vi "Recieve server commands.vi"(8 "error in (no error)":errorcluster, 10 "bytes in":i64, 11 "Control-Client in":refnum<class "Control-Client.lvclass">) -> (0 "error out":errorcluster, 2 "bytes out":i64, 3 "Control-Client out":refnum<class "Control-Client.lvclass">)   [LabVIEW 2019, in "Control-Client.lvclass"]
uses:
  Control-Client.lvclass
  C:/Dev/TRANCON/Classes/GeneralFunctionality/GeneralFunctionality.lvclass
  dependecies/ControlsVIs/Clusters-def/Det-Reply-to-Read.ctl
  dependecies/ControlsVIs/Clusters-def/Def_signals_from_DET.ctl
  Control-Client.lvclass/Control-Client.ctl
  dependecies/ControlsVIs/Clusters-def/ProtypeCommand-CommandUnknown.ctl
  dependecies/ControlsVIs/Clusters-def/DL-Reply-to-Connect-to-Client.ctl
  dependecies/ControlsVIs/Clusters-def/Det-Reply-to-Connect-client.ctl
  dependecies/ControlsVIs/Clusters-def/DAQmx-Reply-Connect-client.ctl
  dependecies/ControlsVIs/Clusters-def/OSc-Reply-Connect-client.ctl
  dependecies/ControlsVIs/Clusters-def/CONTROL-Reply-Allconnect.ctl
  dependecies/ControlsVIs/Clusters-def/CONTROL-Reply-Status-client.ctl
  dependecies/ControlsVIs/Clusters-def/TEST-def.ctl
  dependecies/ControlsVIs/Clusters-def/DLMovedAxis-Com.ctl
  dependecies/ControlsVIs/Clusters-def/ProtypeCommand-DAQmxReply.ctl
  dependecies/ControlsVIs/Clusters-def/DAQmx-ELYSE_pulse_counter.ctl
  dependecies/ControlsVIs/Clusters-def/DAQmx-ELYSE_PumpSpeed.ctl
  dependecies/ControlsVIs/Clusters-def/OSc-Reply-Read.ctl
  dependecies/ControlsVIs/Clusters-def/Message types.ctl
  <vilib>/NI/STM/TCP/Read Message (TCP).vi
  <vilib>/NI/STM/NI STM.lvlib
  Message/Message.lvclass
  Delay Line/DelayLine.lvclass
  Detector/Detector.lvclass
  Control-Server/Control-Server.lvclass
  DAQmxTasks/DAQmxTaskContainer_General/DAQmxTaksContainer_General.lvclass
  Oscilloscope/Oscilloscope.lvclass
  GeneralFunctionality/GeneralFunctionality.lvclass
panel:
  in  "?":T1
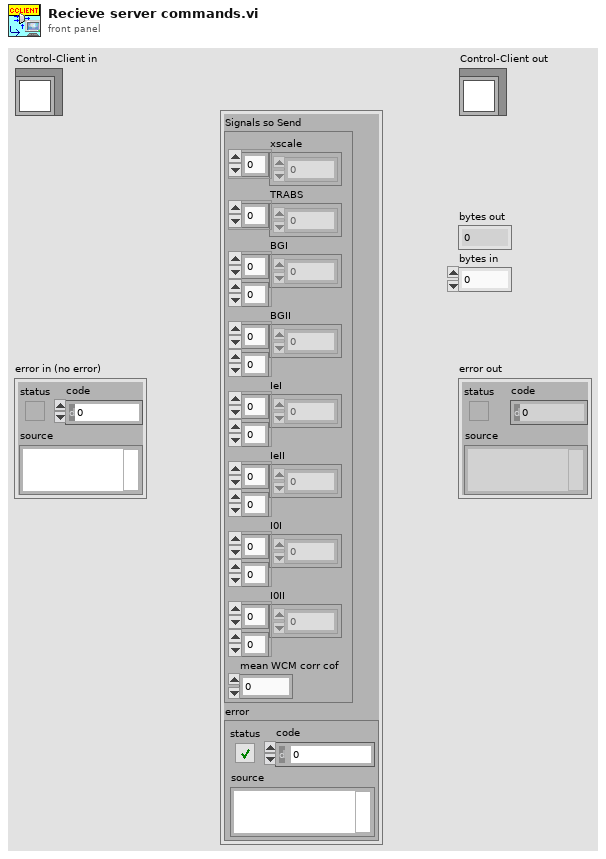
[diagram p1: front panel]
types:
  T1 = typedef "Detector.lvclass/Det-Reply-to-Read.ctl" = cluster{"Signals so Send":T2, "error":errorcluster}
  T2 = typedef "Detector.lvclass/Def_signals_from_DET.ctl" = cluster{"xscale":sgl[], "TRABS":sgl[], "BGI":sgl[][], "BGII":sgl[][], "IeI":sgl[][], "IeII":sgl[][], "I0I":sgl[][], "I0II":sgl[][], "mean WCM corr cof":dbl}
  T3 = typedef "ProtypeCommand-CommandUnknown.ctl" = cluster{"error in (no error)":errorcluster}
  T4 = typedef "DelayLine.lvclass/DL-Reply-to-Connect-to-Client.ctl" = cluster{"on/off":bool, "pos":dbl[], "param":cluster{"min":dbl, "max":dbl, "real pos":dbl}[], "predefine_pos":dbl[][], "error":errorcluster}
  T5 = typedef "Detector.lvclass/Det-Reply-to-Connect-client.ctl" = cluster{"on/off":bool, "calibration":dbl[], "error":errorcluster}
  T6 = typedef "DAQmxTaksContainer_General.lvclass/DAQmx-Reply-Connect-client.ctl" = cluster{"on/off":bool, "RelayKeyHeater/off":bool, "LaserShutter":bool, "AcceleratorShutter":bool, "Power":bool, "Faraday Cup Status":bool, "Pump Start_Stop":bool, "error":errorcluster}
  T7 = typedef "Oscilloscope.lvclass/OSc-Reply-Connect-client.ctl" = cluster{"on/off":bool, "WCM_state":bool, "error":errorcluster}
  T8 = typedef "Control-Server.lvclass/CONTROL-Reply-Allconnect.ctl" = cluster{"On/Off":bool, "error":errorcluster}
  T9 = typedef "Control-Client.lvclass/CONTROL-Reply-Status-client.ctl" = cluster{"DL reply to client":T4, "Det reply to client":cluster{"on/off":bool, "calibration":dbl[], "error out":errorcluster}, "DAQmx reply to client":T6, "OSc reply to CLIENT":T7}
  T10 = typedef "TEST-def.ctl" = cluster{"data":cluster{i32[], dbl[]}[]}
  T11 = typedef "DelayLine.lvclass/DLMovedAxis-Com.ctl" = cluster{"axis":i32, "what was asked":dbl, "where is is now":dbl, "Moved":bool, "error in (no error)":errorcluster}
  T12 = typedef "ProtypeCommand-DAQmxReply.ctl" = cluster{"On/Off":bool, "error out":errorcluster}
  T13 = typedef "DAQmxTaksContainer_General.lvclass/DAQmx-ELYSE_pulse_counter.ctl" = cluster{"# counts":dbl}
  T14 = typedef "DAQmxTaksContainer_General.lvclass/DAQmx-ELYSE_PumpSpeed.ctl" = cluster{"speed, rpm":dbl}
  T15 = typedef "Oscilloscope.lvclass/OSc-Reply-Read.ctl" = cluster{"Data":waveform(dbl)[], "Channels":u16[], "error":errorcluster}
  T16 = typedef "Message types.ctl" = string
  T17 = typedef "NI STM.lvlib/TCP Connection Info.ctl" = cluster{"connection ID":refnum<k5>, "meta data":T18[]}
  T18 = typedef "NI STM.lvlib/MetaDataElement.ctl" = string
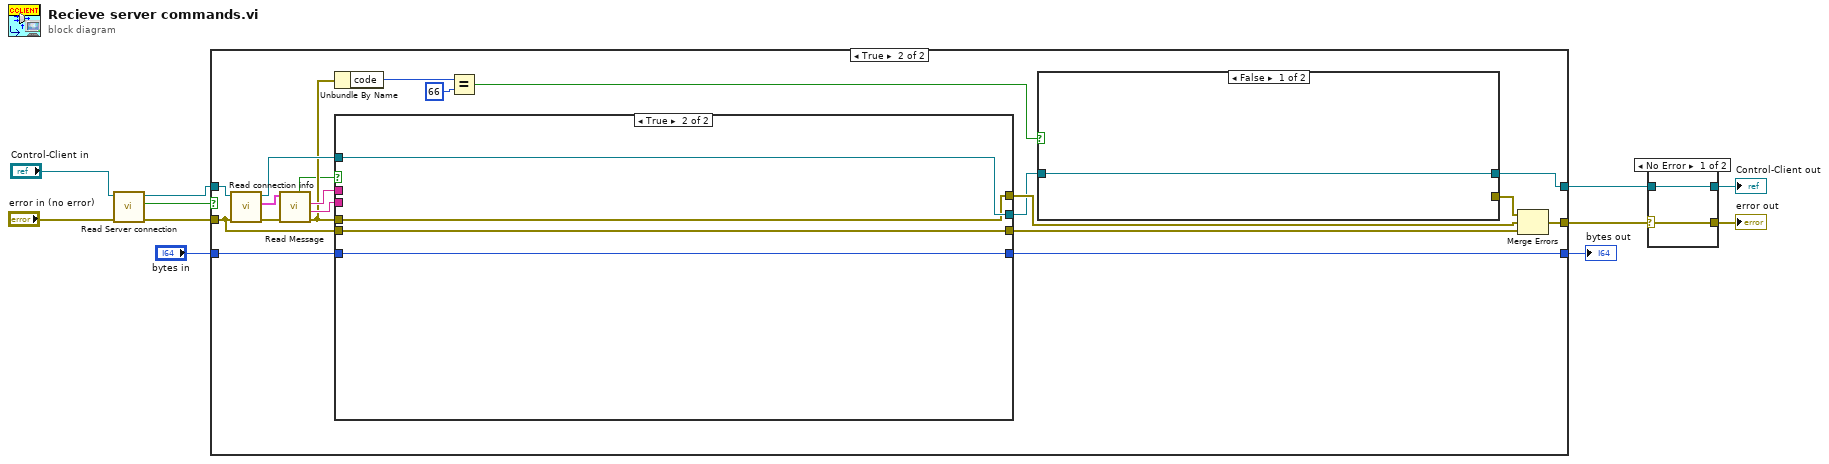
[diagram p0: block diagram]
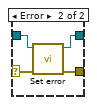
[diagram p2: hidden frame]
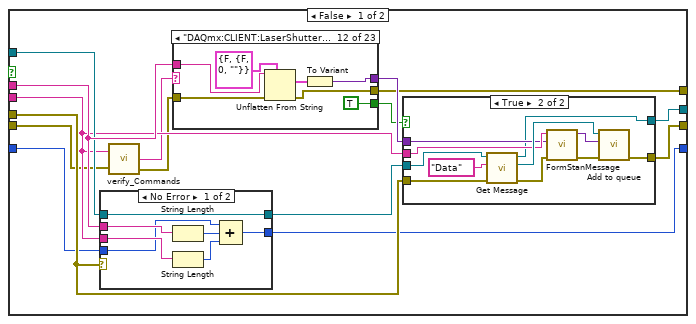
[diagram p4: hidden frame]
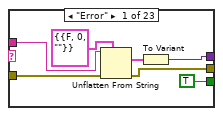
[diagram p6: hidden frame]
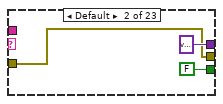
[diagram p7: hidden frame]
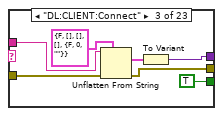
[diagram p8: hidden frame]
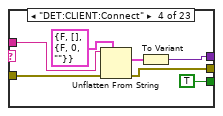
[diagram p9: hidden frame]
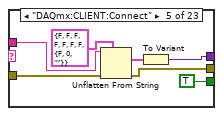
[diagram p10: hidden frame]
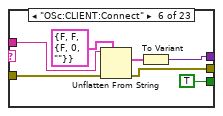
[diagram p11: hidden frame]
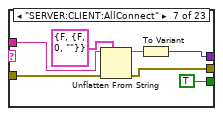
[diagram p12: hidden frame]
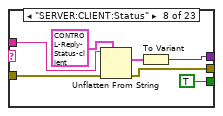
[diagram p13: hidden frame]
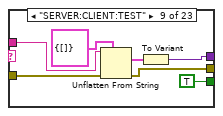
[diagram p14: hidden frame]
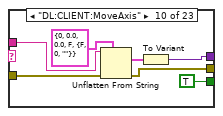
[diagram p15: hidden frame]
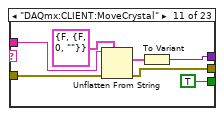
[diagram p16: hidden frame]
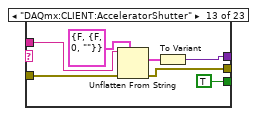
[diagram p17: hidden frame]
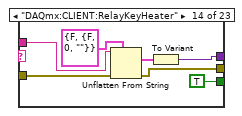
[diagram p18: hidden frame]
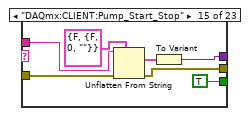
[diagram p19: hidden frame]
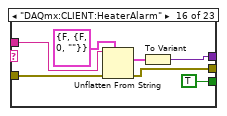
[diagram p20: hidden frame]
diagram:
  n1 = call "Read Server connection.vi"("error in (no error)"="error in (no error)", "Control-Client in"="Control-Client in") -> ("error out"=w4:errorcluster, "Server connection"=w6:bool, "Control-Client out"=w3:refnum<class "Control-Client.lvclass">)  [unwired: 7 in]
  n2 = case shown="True" w6 {
    tunnel: [w14 w26] -> w5
    tunnel: w4 -> [w14 w28]
    tunnel: [w13 w29] -> w2
    tunnel: w3 -> [w13 w23]
    tunnel: "bytes in" -> [w12 w16]
    tunnel: [w12 w15] -> w7
    frame False {
    }
    frame True {
      n3 = call "Read connection info.vi"("error in (no error)"=w28, "Control-Client in"=w23) -> ("error out"=w34:errorcluster, "connection info"=w33:T17, "Control-Client out"=w19:refnum<class "Control-Client.lvclass">)  [unwired: 7 in]
      n4 = call-poly <vilib>:"Read Message.vi"("error in"=w34, "connection info in"=w33) -> ("error out"=w18:errorcluster, "name"=w20:T18, "data string"=w21:string, "timed out?"=w17:bool)  [unwired: 4 in, 2 out]
      n5 = Unbundle By Name(w18) -> ("code"=w32:i32)
      n6 = case shown="True" w17 {
        tunnel: w28 -> [w40 w231]
        tunnel: [w47 w231] -> w27
        tunnel: [w46 w230] -> w25
        tunnel: [w35 w232] -> w22
        tunnel: w21 -> [w45 _]
        tunnel: w20 -> [w42 _]
        tunnel: w19 -> [w44 w232]
        tunnel: w18 -> [w43 w230]
        tunnel: w16 -> [w38 w229]
        tunnel: [w37 w229] -> w15
        frame False {
          n7 = case shown="No Error" w43 {
            tunnel: [w52 w58] -> w36
            tunnel: w45 -> [w56 _]
            tunnel: w42 -> [w54 _]
            tunnel: w44 -> [w52 w58]
            tunnel: w38 -> [w51 w57]
            tunnel: [w50 w57] -> w37
            frame No Error {
              n8 = String Length(string=w56) -> (length=w55:i32)
              n9 = String Length(string=w54) -> (length=w53:i32)
              n10 = Compound Arithmetic op=ADD(w51, w55, w53) -> (w50:i64)
            }
            frame Error {
            }
          }
          n11 = call "verify_Commands.vi"("Command"=w42, "error in"=w40) -> ("Command out"=w41:string, "error out"=w39:errorcluster)  [unwired: 1 out]
          n12 = case shown="\"DAQmx:CLIENT:LaserShutter\"" w41 {
            tunnel: w45 -> [w64 _ w73 w81 w86 w94 w99 w107 w115 w123 w130 w137 w144 w151 w158 w165 w172 w179 w186 w193 w200 w207 w214]
            tunnel: [w61 variant ("Variant") w75 w82 w89 w96 w103 w110 w117 w121 w129 w136 w143 w150 w157 w164 w171 w178 w185 w192 w199 w206 w213] -> w49
            tunnel: [TRUE FALSE TRUE TRUE TRUE TRUE TRUE TRUE TRUE TRUE TRUE TRUE TRUE TRUE TRUE TRUE TRUE TRUE TRUE TRUE TRUE TRUE TRUE] -> w48
            tunnel: w39 -> [w59 w66 w70 w76 w84 w92 w98 w106 w114 w118 w125 w133 w140 w147 w154 w161 w169 w176 w182 w189 w197 w204 w211]
            tunnel: [w60 w66 w69 w77 w83 w91 w97 w105 w113 w119 w126 w132 w139 w146 w153 w160 w168 w175 w181 w188 w196 w203 w210] -> w46
            frame "Error" {
              n13 = Unflatten From String(type=T3 {"error in (no error)"={"status"=FALSE, "code"=0, "source"=""}} ("cluster"), binary string=w64, error in (no error)=w59) -> (value=w62:T3, error out=w60:errorcluster)  [unwired: 2 in, 1 out]
              n14 = To Variant(anything=w62) -> (Variant=w61:variant)
            }
            frame Default {
            }
            frame "DL:CLIENT:Connect" {
              n15 = Unflatten From String(type=T4 {"on/off"=FALSE, "pos"=[], "param"=[], "predefine_pos"=[], "error"={"status"=FALSE, "code"=0, "source"=""}} ("output cluster"), binary string=w73, error in (no error)=w70) -> (value=w71:T4, error out=w69:errorcluster)  [unwired: 2 in, 1 out]
              n16 = To Variant(anything=w71) -> (Variant=w75:variant)
            }
            frame "DET:CLIENT:Connect" {
              n17 = Unflatten From String(type=T5 {"on/off"=FALSE, "calibration"=[], "error"={"status"=FALSE, "code"=0, "source"=""}} ("Cluster"), binary string=w81, error in (no error)=w76) -> (value=w79:T5, error out=w77:errorcluster)  [unwired: 2 in, 1 out]
              n18 = To Variant(anything=w79) -> (Variant=w82:variant)
            }
            frame "DAQmx:CLIENT:Connect" {
              n19 = Unflatten From String(type=T6 {"on/off"=FALSE, "RelayKeyHeater/off"=FALSE, "LaserShutter"=FALSE, "AcceleratorShutter"=FALSE, "Power"=FALSE, "Faraday Cup Status"=FALSE, "Pump Start_Stop"=FALSE, "error"={"status"=FALSE, "code"=0, "source"=""}} ("output cluster"), binary string=w86, error in (no error)=w84) -> (value=w85:T6, error out=w83:errorcluster)  [unwired: 2 in, 1 out]
              n20 = To Variant(anything=w85) -> (Variant=w89:variant)
            }
            frame "OSc:CLIENT:Connect" {
              n21 = Unflatten From String(type=T7 {"on/off"=FALSE, "WCM_state"=FALSE, "error"={"status"=FALSE, "code"=0, "source"=""}} ("output cluster"), binary string=w94, error in (no error)=w92) -> (value=w93:T7, error out=w91:errorcluster)  [unwired: 2 in, 1 out]
              n22 = To Variant(anything=w93) -> (Variant=w96:variant)
            }
            frame "SERVER:CLIENT:AllConnect" {
              n23 = Unflatten From String(type=T8 {"On/Off"=FALSE, "error"={"status"=FALSE, "code"=0, "source"=""}} ("output cluster"), binary string=w99, error in (no error)=w98) -> (rest of the binary string=w101:string, error out=w97:errorcluster)  [unwired: 2 in, 1 out]
              n24 = To Variant(anything=w101) -> (Variant=w103:variant)
            }
            frame "SERVER:CLIENT:Status" {
              n25 = Unflatten From String(type=T9 {"DL reply to client"={"on/off"=FALSE, "pos"=[], "param"=[], "predefine_pos"=[], "error"={"status"=FALSE, "code"=0, "source"=""}}, "Det reply to client"={"on/off"=FALSE, "calibration"=[], "error out"={"status"=FALSE, "code"=0, "source"=""}}, "DAQmx reply to client"={"on/off"=FALSE, "RelayKeyHeater/off"=FALSE, "LaserShutter"=FALSE, "AcceleratorShutter"=FALSE, "Power"=FALSE, "Faraday Cup Status"=FALSE, "Pump Start_Stop"=FALSE, "error"={"status"=FALSE, "code"=0, "source"=""}}, "OSc reply to CLIENT"={"on/off"=FALSE, "WCM_state"=FALSE, "error"={"status"=FALSE, "code"=0, "source"=""}}} ("output cluster"), binary string=w107, error in (no error)=w106) -> (value=w104:T9, error out=w105:errorcluster)  [unwired: 2 in, 1 out]
              n26 = To Variant(anything=w104) -> (Variant=w110:variant)
            }
            frame "SERVER:CLIENT:TEST" {
              n27 = Unflatten From String(type=T10 {"data"=[]} ("output cluster"), binary string=w115, error in (no error)=w114) -> (value=w112:T10, error out=w113:errorcluster)  [unwired: 2 in, 1 out]
              n28 = To Variant(anything=w112) -> (Variant=w117:variant)
            }
            frame "DL:CLIENT:MoveAxis" {
              n29 = Unflatten From String(type=T11 {"axis"=0, "what was asked"=0.0, "where is is now"=0.0, "Moved"=FALSE, "error in (no error)"={"status"=FALSE, "code"=0, "source"=""}} ("cluster"), binary string=w123, error in (no error)=w118) -> (value=w124:T11, error out=w119:errorcluster)  [unwired: 2 in, 1 out]
              n30 = To Variant(anything=w124) -> (Variant=w121:variant)
            }
            frame "DAQmx:CLIENT:MoveCrystal" {
              n31 = Unflatten From String(type=T12 {"On/Off"=FALSE, "error out"={"status"=FALSE, "code"=0, "source"=""}} ("output cluster"), binary string=w130, error in (no error)=w125) -> (value=w131:T12, error out=w126:errorcluster)  [unwired: 2 in, 1 out]
              n32 = To Variant(anything=w131) -> (Variant=w129:variant)
            }
            frame "DAQmx:CLIENT:LaserShutter" {
              n33 = Unflatten From String(type=T12 {"On/Off"=FALSE, "error out"={"status"=FALSE, "code"=0, "source"=""}} ("output cluster"), binary string=w137, error in (no error)=w133) -> (value=w138:T12, error out=w132:errorcluster)  [unwired: 2 in, 1 out]
              n34 = To Variant(anything=w138) -> (Variant=w136:variant)
            }
            frame "DAQmx:CLIENT:AcceleratorShutter" {
              n35 = Unflatten From String(type=T12 {"On/Off"=FALSE, "error out"={"status"=FALSE, "code"=0, "source"=""}} ("output cluster"), binary string=w144, error in (no error)=w140) -> (value=w145:T12, error out=w139:errorcluster)  [unwired: 2 in, 1 out]
              n36 = To Variant(anything=w145) -> (Variant=w143:variant)
            }
            frame "DAQmx:CLIENT:RelayKeyHeater" {
              n37 = Unflatten From String(type=T12 {"On/Off"=FALSE, "error out"={"status"=FALSE, "code"=0, "source"=""}} ("output cluster"), binary string=w151, error in (no error)=w147) -> (value=w152:T12, error out=w146:errorcluster)  [unwired: 2 in, 1 out]
              n38 = To Variant(anything=w152) -> (Variant=w150:variant)
            }
            frame "DAQmx:CLIENT:Pump_Start_Stop" {
              n39 = Unflatten From String(type=T12 {"On/Off"=FALSE, "error out"={"status"=FALSE, "code"=0, "source"=""}} ("output cluster"), binary string=w158, error in (no error)=w154) -> (value=w159:T12, error out=w153:errorcluster)  [unwired: 2 in, 1 out]
              n40 = To Variant(anything=w159) -> (Variant=w157:variant)
            }
            frame "DAQmx:CLIENT:HeaterAlarm" {
              n41 = Unflatten From String(type=T12 {"On/Off"=FALSE, "error out"={"status"=FALSE, "code"=0, "source"=""}} ("output cluster"), binary string=w165, error in (no error)=w161) -> (value=w166:T12, error out=w160:errorcluster)  [unwired: 2 in, 1 out]
              n42 = To Variant(anything=w166) -> (Variant=w164:variant)
            }
            frame "DAQmx:CLIENT:ELYSE_pulse_counter" {
              n43 = Unflatten From String(type=T13 {"# counts"=0.0} ("OSc:Read"), binary string=w172, error in (no error)=w169) -> (value=w173:T13, error out=w168:errorcluster)  [unwired: 2 in, 1 out]
              n44 = To Variant(anything=w173) -> (Variant=w171:variant)
            }
            frame "DAQmx:CLIENT:PumpSpeed" {
              n45 = Unflatten From String(type=T14 {"speed, rpm"=0.0} ("OSc:Read"), binary string=w179, error in (no error)=w176) -> (value=w180:T14, error out=w175:errorcluster)  [unwired: 2 in, 1 out]
              n46 = To Variant(anything=w180) -> (Variant=w178:variant)
            }
            frame "DAQmx:CLIENT:PowerStatus" {
              n47 = Unflatten From String(type=T12 {"On/Off"=FALSE, "error out"={"status"=FALSE, "code"=0, "source"=""}} ("output cluster"), binary string=w186, error in (no error)=w182) -> (value=w187:T12, error out=w181:errorcluster)  [unwired: 2 in, 1 out]
              n48 = To Variant(anything=w187) -> (Variant=w185:variant)
            }
            frame "DAQmx:CLIENT:FaradayCupStatus" {
              n49 = Unflatten From String(type=T12 {"On/Off"=FALSE, "error out"={"status"=FALSE, "code"=0, "source"=""}} ("output cluster"), binary string=w193, error in (no error)=w189) -> (value=w194:T12, error out=w188:errorcluster)  [unwired: 2 in, 1 out]
              n50 = To Variant(anything=w194) -> (Variant=w192:variant)
            }
            frame "DAQmx:CLIENT:Status" {
              n51 = Unflatten From String(type=T6 {"on/off"=FALSE, "RelayKeyHeater/off"=FALSE, "LaserShutter"=FALSE, "AcceleratorShutter"=FALSE, "Power"=FALSE, "Faraday Cup Status"=FALSE, "Pump Start_Stop"=FALSE, "error"={"status"=FALSE, "code"=0, "source"=""}} ("output cluster"), binary string=w200, error in (no error)=w197) -> (value=w201:T6, error out=w196:errorcluster)  [unwired: 2 in, 1 out]
              n52 = To Variant(anything=w201) -> (Variant=w199:variant)
            }
            frame "DET:CLIENT:Read" {
              n53 = Unflatten From String(type="?", binary string=w207, error in (no error)=w204) -> (value=w208:T1, error out=w203:errorcluster)  [unwired: 2 in, 1 out]
              n54 = To Variant(anything=w208) -> (Variant=w206:variant)
            }
            frame "OSc:CLIENT:Read" {
              n55 = Unflatten From String(type=T15 {"Data"=[], "Channels"=[], "error"={"status"=FALSE, "code"=0, "source"=""}} ("Cluster"), binary string=w214, error in (no error)=w211) -> (value=w215:T15, error out=w210:errorcluster)  [unwired: 2 in, 1 out]
              n56 = To Variant(anything=w215) -> (Variant=w213:variant)
            }
          }
          n57 = case shown="True" w48 {
            tunnel: [w217 w228] -> w47
            tunnel: w42 -> [_ w223]
            tunnel: w49 -> [_ w222]
            tunnel: w43 -> [w217 w225]
            tunnel: w36 -> [w216 w224]
            tunnel: [w216 w218] -> w35
            frame False {
            }
            frame True {
              n58 = call "Get Message.vi"("error in (no error)"=w225, "Message type"=T16 "Data", "GeneralFunctionality en entrée"=w224) -> ("error out"=w220:errorcluster, "Message.lvclass"=w226:refnum<class "Message.lvclass">, "GeneralFunctionality en sortie"=w218:refnum<class "Control-Client.lvclass">)  [unwired: 6 in]
              n59 = call "FormStanMessage.vi"("error in"=w220, "data"=w222, "Command"=w223) -> ("error out"=w219:errorcluster, "message"=w221:variant)  [unwired: 7 in]
              n60 = call "Add to queue.vi"("error in (no error)"=w219, "Data"=w221, "Message in"=w226) -> ("error out"=w228:errorcluster)  [unwired: 7 in, 1 out]
            }
          }
        }
        frame True {
        }
      }
      n61 = Equal?(x=w32, y=66) -> (x = y?=w30:bool)
      n62 = case shown="False" w30 {
        selector: w30 -> [_ w244]
        tunnel: w22 -> [w233 w234]
        tunnel: [w233 w241] -> w29
        tunnel: [_ w235] -> w24
        frame False {
        }
        frame True {
          n63 = Type Cast(x=w244) -> (*(type *) &x=w237:string)  [unwired: 1 in]
          n64 = call "Get Message.vi"("Message type"=T16 "Data", "GeneralFunctionality en entrée"=w234) -> ("error out"=w238:errorcluster, "Message.lvclass"=w247:refnum<class "Message.lvclass">, "GeneralFunctionality en sortie"=w243:refnum<class "Control-Client.lvclass">)  [unwired: 7 in]
          n65 = Bundle By Name(cluster=w243, "Server connection"=FALSE) -> (w241:refnum<class "Control-Client.lvclass">)
          n66 = call "FormStanMessage.vi"("error in"=w238, "data"=w237, "Command"="ConnectionBreak" ("command name")) -> ("error out"=w239:errorcluster, "message"=w240:variant)  [unwired: 7 in]
          n67 = To Variant(anything=w240) -> (Variant=w245:variant)
          n68 = call "Add to queue.vi"("error in (no error)"=w239, "Data"=w245, "Message in"=w247) -> ("error out"=w235:errorcluster)  [unwired: 7 in, 1 out]
        }
      }
      n69 = Merge Errors(w24, w25, w27) -> (w26:errorcluster)
    }
  }
  "bytes out" <- w7
  n70 = case shown="No Error" w5 {
    selector: w5 -> [w249 w251]
    tunnel: w2 -> [w248 w253]
    tunnel: [w249 w252] -> w10
    tunnel: [w248 w250] -> w1
    frame No Error {
    }
    frame Error {
      n71 = call "Set error.vi"("error in (no error)"=w251, "Control-Client in"=w253) -> ("error out"=w252:errorcluster, "Control-Client out"=w250:refnum<class "Control-Client.lvclass">)  [unwired: 8 in]
    }
  }
  "error out" <- w10
  "Control-Client out" <- w1
